vi "Is Ref Valid.vi"(8 "error in (no error)":errorcluster, 11 "Class Reference Control in":refnum<class "Class Reference Control.lvclass">) -> (0 "error out":errorcluster, 2 "Refnum Valid?":bool, 3 "Class Reference Control out":refnum<class "Class Reference Control.lvclass">)   [LabVIEW 2016, in "Class Reference Control.lvclass"]
uses:
  Class Reference Control.lvclass
  Class Reference Control.lvclass/Class Reference Control.ctl
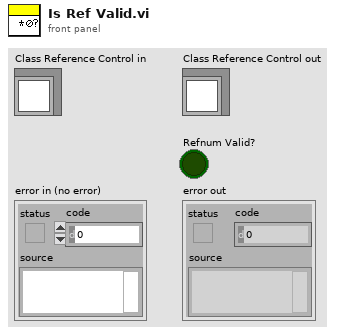
[diagram p1: front panel]
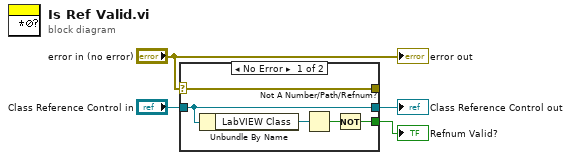
[diagram p0: block diagram]
diagram:
  n1 = case shown="No Error" "error in (no error)" {
    selector: "error in (no error)" -> [w9 w11]
    tunnel: [w9 w11] -> _
    tunnel: [w8 w10] -> w2
    tunnel: "Class Reference Control in" -> [w8 w10]
    tunnel: [w5 _] -> w1
    frame No Error {
      n2 = Unbundle By Name(w8) -> ("LabVIEW Class"=w7:refnum<vi>)
      n3 = Not A Number/Path/Refnum?(number/path/refnum=w7) -> (NaN/Path/Refnum?=w6:bool)
      n4 = Not(x=w6) -> (.not. x?=w5:bool)
    }
    frame Error {
    }
  }
  "Class Reference Control out" <- w2
  "Refnum Valid?" <- w1
  "error out" <- "error in (no error)"
